vi "Verbose Style.vi"() -> (0 "Message Formatting":T1={"Font"="Consolas", "Text Color"=enum."Gray", "Text Background Color"=enum."White", "Text Style"=enum."Italic", "Font Size (Points)"=10.0, "Text Alignment"=0} {"Text Alignment" items=["Left", "Right", "Center"]})   [LabVIEW 2019, in "Rich Text Box.lvlib"]
uses:
  Rich Text Box.lvlib
  Text Formatting.ctl
  Text Colors.ctl
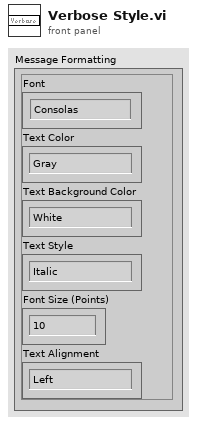
[diagram p1: front panel]
types:
  T1 = typedef "Rich Text Box.lvlib/Text Formatting.ctl" = cluster{"Font":string, "Text Color":T2, "Text Background Color":T2, "Text Style":enum16{"Regular", "Bold", "Italic", "Underline", "Strikeout"}, "Font Size (Points)":dbl, "Text Alignment":i32}
  T2 = typedef "Rich Text Box.lvlib/Text Colors.ctl" = enum16{"Unchanged", "Black", "Blue", "Gray", "Green", "Red", "White"}
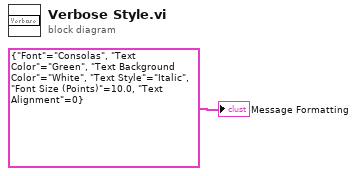
[diagram p0: block diagram]
diagram:
  "Message Formatting" <- T1 {"Font"="Consolas", "Text Color"=enum."Green", "Text Background Color"=enum."White", "Text Style"=enum."Italic", "Font Size (Points)"=10.0, "Text Alignment"=0} ("Default Text Formatting")
